vi "ball_demo_finished.vi"() -> ()   [LabVIEW 2011]
uses:
  <vilib>/imath/engines/lvmath2/RunTimeEngine/ErrorHandling/NIMS_Finalize Error.vi
  <vilib>/imath/engines/lvmath2/RunTimeEngine/CommandStatement/NIMS_CommandStatement_MaskErr.vi
  <vilib>/imath/engines/lvmath2/RunTimeEngine/VariableToken/NIMS_VariableToken_CondDefined.vi
  <instcachedir>/0/NIMS_VariableToken_CondDefined_D30D2F4D3CE04567BC79CC35D27951F7.lvgen/NIMS_VariableToken_CondDefined_D30D2F4D3CE04567BC79CC35D27951F7_003.vi
  <vilib>/imathl/engines/lvmath/Functions/Error Handling/Create Error.vi
  <vilib>/imath/engines/lvmath/Functions/Error Handling/MergeErrorsWrapper.vi
  <vilib>/imath/engines/lvmath2/RunTimeEngine/NodeEndStatement/NIMS_NodeEndStatement_Output.vi
  <instcachedir>/0/NIMS_NodeEndStatement_Output_53EC0D466D134D7ABD903AC30B43404B.lvgen/NIMS_NodeEndStatement_Output_53EC0D466D134D7ABD903AC30B43404B_005.vi
  <vilib>/imath/engines/lvmath2/RunTimeEngine/BuiltInFunctions/abs/NIMS_abs(signed).vi
  <instcachedir>/0/NIMS_abs(signed)_C4FCB8E6058B49B797C7C8D53CA5F6EC.lvgen/NIMS_abs(signed)_C4FCB8E6058B49B797C7C8D53CA5F6EC_000.vi
  <vilib>/imath/engines/lvmath2/RunTimeEngine/CommandStatement/MC_CommandStatement_break.vi
  <vilib>/imath/engines/lvmath2/RunTimeEngine/VariableToken/NIMS_VariableToken_CondDefinedDefinedByReplace.vi
  <instcachedir>/0/NIMS_VariableToken_CondDefinedDefinedByReplace_D162CFFC24174562A9FEA619A91E1A56.lvgen/NIMS_VariableToken_CondDefinedDefinedByReplace_D162CFFC24174562A9FEA619A91E1A56_002.vi
  <vilib>/imath/engines/lvmath2/RunTimeEngine/ReplaceToken/NIMS_Replace - Check Linear.vi
  <instcachedir>/0/NIMS_Replace - Check Linear_276AD648BD064726893CCF9ED6E2A728.lvgen/NIMS_Replace - Check Linear_276AD648BD064726893CCF9ED6E2A728_001.vi
  <vilib>/imath/engines/lvmath2/RunTimeEngine/ReplaceToken/NIMS_Replace - Size Check _(_)=S.vi
  <instcachedir>/0/NIMS_Replace - Size Check _(_)=S_9ABE7AF2D26C43EAA05192D5C1E6C624.lvgen/NIMS_Replace - Size Check _(_)=S_9ABE7AF2D26C43EAA05192D5C1E6C624_000.vi
  <vilib>/imath/engines/lvmath2/RunTimeEngine/ReplaceToken/NIMS_Replace - V(S)=S.vi
  <instcachedir>/0/NIMS_Replace - V(S)=S_16B13A4565AB46F59881314645612498.lvgen/NIMS_Replace - V(S)=S_16B13A4565AB46F59881314645612498_000.vi
panel:
  out "MATLAB":cluster{dbl[], dbl[]}[](graph)
  in  "stop":bool
  in  "Initial velocity":dbl(knob) scale=-15.0..15.0
  in  "Coefficient of Restitution":dbl(knob)=1.0 scale=0.0..1.5
  in  "Initial height":dbl(knob)=5.0 scale=5.0..20.0
  out "LabVIEW":cluster{dbl[], dbl[]}[](graph)
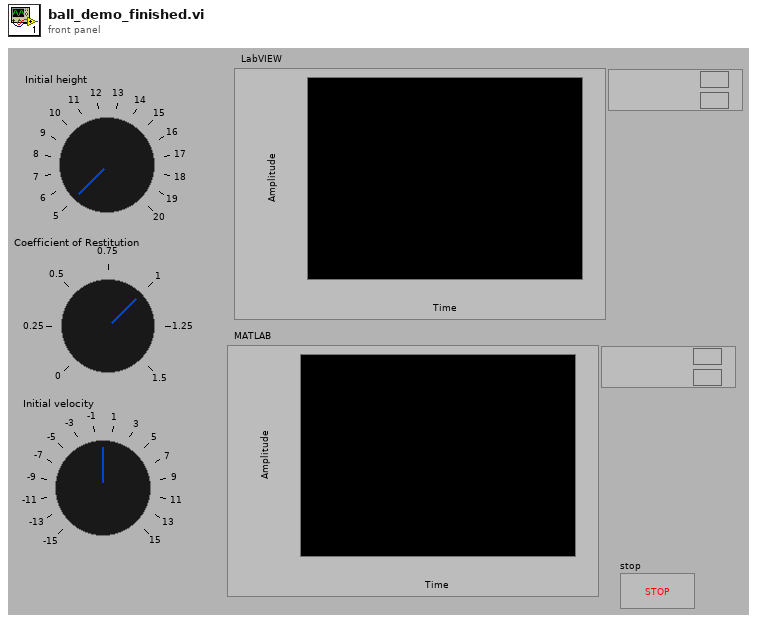
[diagram p1: front panel]
types:
  T1 = cluster{"actual_time":dbl[], "actual_height":dbl[]}
  T2 = cluster{"actual_time":dbl[], "actual_velocity":dbl[]}
  T3 = cluster{"actual_time":dbl[], "actual_velocity":dbl[]}[]
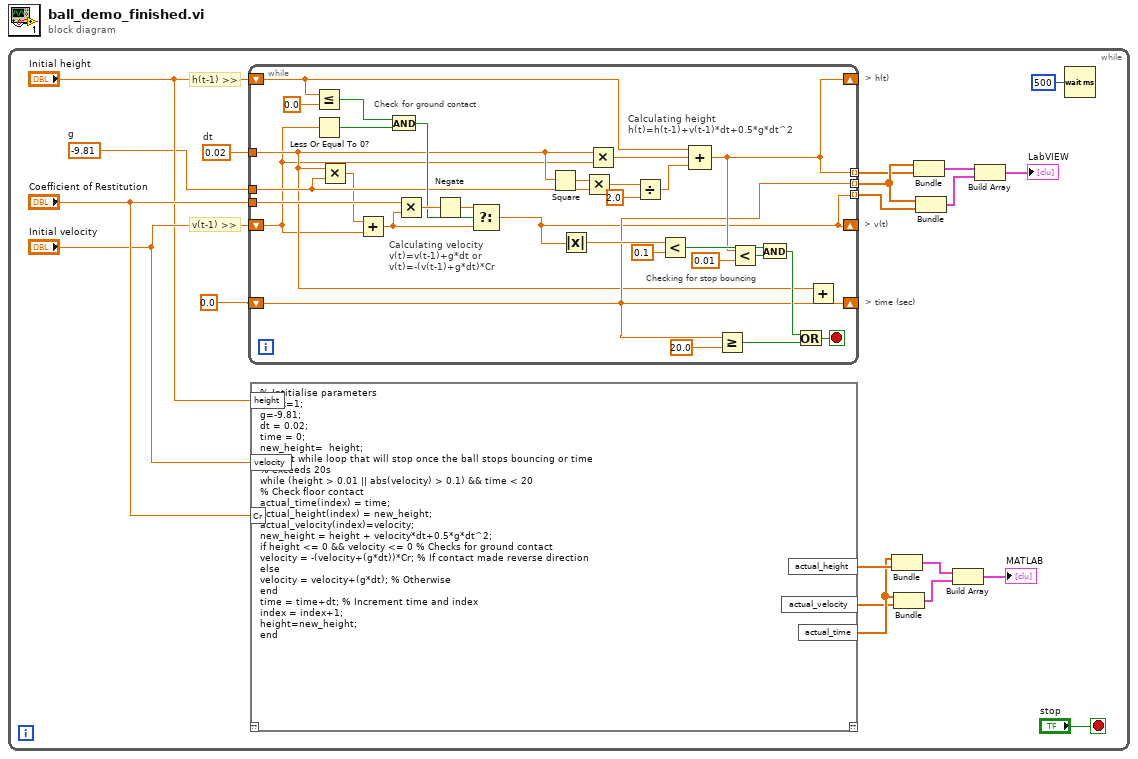
[diagram p0: block diagram]
diagram:
  n1 = while {
    stop <- "stop" stop-if-true
    w7 = 0.02  # dt
    w8 = -9.81  # g
    # "> v(t)"
    # "v(t-1) >>"
    # "h(t-1) >>"
    # "> h(t)"
    # "> time (sec)"
    n2 = while {
      tunnel: w7 -> [w312]
      tunnel: w8 -> [w320]
      shift-right: [w311] -> _
      shift-left: "Initial velocity" -> [w310]
      shift-right: [w316] -> _
      shift-left: "Initial height" -> [w331]
      tunnel: "Coefficient of Restitution" -> [w322]
      shift-right: [w314] -> _
      shift-left: 0.0 ("time") -> [w313]
      tunnel: [w316] -> w19 mode=indexing
      tunnel: [w311] -> w18 mode=indexing
      tunnel: [w313] -> w20 mode=indexing
      stop <- w327 stop-if-true
      # "Checking for stop bouncing"
      # "Calculating velocity\nv(t)=v(t-1)+g*dt or\nv(t)=-(v(t-1)+g*dt)*Cr"
      # "Check for ground contact"
      # "Calculating height\nh(t)=h(t-1)+v(t-1)*dt+0.5*g*dt^2"
      n3 = Less Or Equal?(x=w331, y=0.0) -> (x <= y?=w334:bool)
      n4 = Less Or Equal To 0?(x=w310) -> (x <= 0?=w333:bool)
      n5 = Multiply(x=w312, y=w320) -> (x*y=w309:dbl)
      n6 = Add(x=w309, y=w310) -> (x+y=w308:dbl)
      n7 = And(x=w334, y=w333) -> (x .and. y?=w332:bool)
      n8 = Multiply(x=w322, y=w308) -> (x*y=w336:dbl)
      n9 = Negate(x=w336) -> (-x=w335:dbl)
      n10 = Select(t=w335, s=w332, f=w308) -> (s? t:f=w311:dbl)
      n11 = Square(x=w312) -> (x^2=w321:dbl)
      n12 = Absolute Value(x=w311) -> (abs(x)=w329:dbl)
      n13 = Multiply(x=w321, y=w320) -> (x*y=w319:dbl)
      n14 = Multiply(x=w312, y=w310) -> (x*y=w338:dbl)
      n15 = Divide(x=w319, y=2.0) -> (x/y=w317:dbl)
      n16 = Less?(x=w329, y=0.1) -> (x < y?=w323:bool)
      n17 = Compound Arithmetic op=ADD(w331, w338, w317) -> (w316:dbl)
      n18 = Greater Or Equal?(x=w313, y=20.0 ("x")) -> (x >= y?=w326:bool)
      n19 = Less?(x=w316, y=0.01) -> (x < y?=w324:bool)
      n20 = And(x=w323, y=w324) -> (x .and. y?=w325:bool)
      n21 = Or(x=w325, y=w326) -> (x .or. y?=w327:bool)
      n22 = Add(x=w312, y=w313) -> (x+y=w314:dbl)
    }
    n23 = mathscript code="% Intitialise parameters\nindex=1;\ng=-9.81;\ndt = 0.02;\ntime = 0;\nnew_height=  height;\n% start while loop that will stop once the ball stops bouncing or time\n% exceeds 20s\nwhile (height > 0.01 || abs(velocity) > 0.1) && time < 20\n% Check floor contact\nactual_time(index) = time;\nactual_height(index) = new_height; \nactual_velocity(index)=velocity;\nnew_height = height + velocity*dt+0.5*g*dt^2;\nif height <= 0 && velocity <= 0 % Checks for ground contact\nvelocity = -(velocity+(g*dt))*Cr; % If contact made reverse direction \nelse\nvelocity = velocity+(g*dt); % Otherwise\nend\ntime = time+dt; % Increment time and index\nindex = index+1;\nheight=new_height;\nend"("Cr"="Coefficient of Restitution", "height"="Initial height", "velocity"="Initial velocity") -> ("actual_height"=w3:dbl[], "actual_velocity"=w1:dbl[], "actual_time"=w2:dbl[])  [unwired: 1 in, 1 out]
    n24 = Bundle("actual_time"=w2, "actual_height"=w3) -> (w6:T1)  [unwired: 1 in]
    n25 = Bundle("actual_time"=w2, "actual_velocity"=w1) -> (w5:T2)  [unwired: 1 in]
    n26 = Bundle(w20, w19) -> (w17:cluster{dbl[], dbl[]})  [unwired: 1 in]
    n27 = Bundle(w20, w18) -> (w16:cluster{dbl[], dbl[]})  [unwired: 1 in]
    n28 = Build Array(w6, w5) -> (→"MATLAB":T3)
    n29 = Build Array(w17, w16) -> (→"LabVIEW":cluster{dbl[], dbl[]}[])
    n30 = Wait (ms)(milliseconds to wait=u32 500) -> ()  [unwired: 1 out]
  }
